vi "Measurement Logic.vi"() -> ()   [LabVIEW 2022 SP3, in "Frequency Response.lvlib"]
uses:
  Frequency Response.lvlib
  <vilib>/Plug-In SDKs/Measurements/Measure Call Context/Measure Call Context.lvclass
  Measurement Configuration.ctl
  shared/controls/sweep profile.ctl
  Measurement Results.ctl
  <vilib>/PDM Acquisition Toolkit/host/Classes/Tasks/PDM Tasks/Controls/Acquisition Mode.ctl
  <vilib>/PDM Acquisition Toolkit/shared/controls/clock mode.ctl
  shared/measurements/controls/units settings - mic.ctl
  shared/measurements/controls/measurement units.ctl
  shared/measurements/controls/single tone microphone measurement settings.ctl
  <vilib>/addons/_NISVFA/_Generation/Signal Generation/SV Signal/SV Signal.lvclass/SV Signal.ctl
  <vilib>/addons/_NISVFA/_Generation/Signal Generation/SV Discrete Sweep/SV Discrete Sweep.lvclass/SV Discrete Sweep.ctl
  <vilib>/addons/_NISVFA/_Generation/Signal Generation/SV Signal/Write Leading Synchronization Pulse Enable.vi
  <vilib>/addons/_NISVFA/_Generation/Signal Generation/SV Signal/Write Synchronization Pulse Duration.vi
  <vilib>/addons/_NISVFA/_Generation/Signal Generation/SV Signal/Write Synchronization Pulse Level.vi
  <vilib>/addons/_NISVFA/_Generation/Signal Generation/SV Signal/Write Synchronization Pulse Type.vi
  <vilib>/addons/_NISVFA/_Generation/Signal Generation/SV Signal/Read Total Samples.vi
  shared/measurements/sound and vibration/Align Waveforms by Leading Sync Pulse.vi
  <vilib>/addons/_NISVFA/_Generation/Signal Generation/SV Signal/Read Synchronization Pulse Waveform.vi
  <vilib>/addons/_NISVFA/_Shared subVIs/Common/svc_Check for Waveform Parameter Continuity (N Ch).vi
  Program Files/NI/LVAddons/nisvt/1/examples/Sound and Vibration/Audio Measurements/subVIs/sv_Append Virtual Reference.vi
  <vilib>/addons/_NISVFA/_Generation/Signal Generation/SV Discrete Sweep/Read Frequencies and Amplitudes.vi
  <vilib>/addons/_NISVFA/_Generation/Signal Generation/SV Signal/Calculate Number of Remaining Samples.vi
  shared/measurements/sound and vibration/Measure Delay for Active and Idle Channels.vi
  <vilib>/addons/_NISVFA/_Generation/Signal Generation/SV Signal/Read Leading Synchronization Pulse Enable.vi
  <vilib>/addons/_NISVFA/_Generation/Signal Generation/SV Signal/Read Trailing Synchronization Pulse Enable.vi
  <vilib>/addons/_NISVFA/_Shared subVIs/Common/svc_Check for Waveform Parameter Continuity (no state).vi
  <vilib>/addons/_NISVFA/_Shared subVIs/Common/sv_Get NI Property Name String.vi
  <vilib>/addons/Sound and Vibration/svt_Calibration/SV Measure Delay and Polarity and Coherence (Nx1).vi
  Program Files/NI/LVAddons/nisvt/1/examples/Sound and Vibration/Audio Measurements/subVIs/sv_Assign Delay to Idle Channels.vi
  <vilib>/addons/_NISVFA/_Shared subVIs/Common/svc_Get SV Channel Info.vi
  <vilib>/addons/Sound and Vibration/svt_Calibration/SV Measure Delay and Polarity and Coherence.vi
  <vilib>/addons/_NISVFA/_Shared subVIs/Common/svc_Unit Label to Engineering Units.vi
  <vilib>/addons/_NISVFA/_Shared subVIs/Common/svc_Engineering Units to Unit Label.vi
  <vilib>/Analysis/_algsub.llb/Vector Norm.vi
  <vilib>/Analysis/_algsub.llb/Real Vector Norm.vi
  <vilib>/addons/_NISVFA/_Shared subVIs/Common/SV Get Data Subset.vi
  <vilib>/addons/_NISVFA/_Shared subVIs/Common/svc_Get Array Subset (Index).vi
  <vilib>/addons/_NISVFA/_Shared subVIs/Common/svc_Coerce Index and Length.vi
  <vilib>/addons/_NISVFA/_Shared subVIs/Common/svc_Conditional Merge Error.vi
  <vilib>/addons/_NISVFA/_Generation/Signal Generation/SV Discrete Sweep/SV Discrete Sweep.lvclass
  C:/Program Files/NI/LVAddons/nisvt/1/vi.lib/addons/_NISVFA/_Generation/Signal Generation/SV Signal/SV Signal.lvclass
  C:/Program Files/NI/LVAddons/nisvt/1/vi.lib/addons/_NISVFA/_Generation/Signal Generation/SV Function/SV Function.lvclass
  <vilib>/addons/_NISVFA/_Generation/Signal Generation/SV Signal/Write Ramp Parameters.vi
  <vilib>/addons/_NISVFA/_Generation/Signal Generation/SV Signal/Write Measurement Duration.vi
  <vilib>/addons/_NISVFA/_Generation/Signal Generation/SV Function/Write Measurement Cycles.vi
  <vilib>/addons/_NISVFA/_Generation/Signal Generation/SV Signal/Write Pre-Measurement Settling Duration.vi
  <vilib>/addons/_NISVFA/_Generation/Signal Generation/SV Function/Write Pre-Measurement Settling Cycles.vi
  <vilib>/addons/_NISVFA/_Generation/Signal Generation/SV Signal/Write Sample Rate.vi
  <vilib>/addons/_NISVFA/_Generation/Signal Generation/SV Signal/Read Sample Rate.vi
  <vilib>/addons/_NISVFA/_Generation/Signal Generation/SV Signal/Read Generation State.vi
  <vilib>/addons/_NISVFA/_Generation/Signal Generation/SV Signal/Read System Timing Model.vi
  <vilib>/DAQmx/configure/timing.llb/DAQmx Timing (Sample Clock).vi
  <vilib>/DAQmx/miscellaneous.llb/DAQmx Fill In Error Info.vi
  <vilib>/addons/_NISVFA/_Generation/Signal Generation/SV Signal/Write System Timing Model.vi
  <vilib>/addons/_NISVFA/_Shared subVIs/Data Objects/Waveforms (DBL)/SV Read Newest Data.vi
  <vilib>/measure/maresamp.llb/Resample Waveforms (single shot).vi
  <vilib>/measure/maresamp.llb/Resample Waveform (single shot).vi
  <vilib>/addons/_NISVFA/_Shared subVIs/Common/svc_Check dt for Equal Sample Rates.vi
  <vilib>/Waveform/TSOps.llb/Timestamp Subtract.vi
  <vilib>/Analysis/2dsp.llb/CrossCorrelation.vi
  <vilib>/Analysis/2dsp.llb/1D Cross Correlation (DBL).vi
  <vilib>/addons/_NISVFA/_Shared subVIs/Common/svc_Fit Quadratic to Max Three Points in Array.vi
  <vilib>/Utility/error.llb/Error Cluster From Error Code.vi
  <vilib>/addons/_NISVFA/_Shared subVIs/Common/svc_Caller VI Returned in Error Source.vi
  <vilib>/addons/_NISVFA/_Shared subVIs/Common/SV Remove Delays (1,N) from Waveforms (N Ch) (DBL).vi
  <vilib>/addons/_NISVFA/_Shared subVIs/Common/SV Remove Delays from Waveforms.vi
  <vilib>/addons/_NISVFA/_Generation/Signal Generation/SV Signal/SV Signal.lvclass
  <vilib>/DAQmx/read.llb/DAQmx Read (Analog 1D Wfm NChan NSamp).vi
  <vilib>/addons/_NISVFA/_Generation/Signal Generation/SV Discrete Sweep/Configure Frequency Sweep at Constant Amplitude.vi
  <vilib>/addons/_NISVFA/_Shared subVIs/Data Objects/Waveforms (DBL)/SV Read Next Measurement Data.vi
  <vilib>/DAQmx/write.llb/DAQmx Write (Analog Wfm 1Chan NSamp).vi
  <vilib>/DAQmx/create/channels.llb/DAQmx Create Channel (AO-Voltage-Basic).vi
  <vilib>/DAQmx/configure/trigger.llb/DAQmx Start Trigger (Digital Edge).vi
  <vilib>/DAQmx/configure/events/hardwareSignals.llb/DAQmx Export Signal (Most Signals).vi
  <vilib>/DAQmx/create/channels.llb/DAQmx Create Channel (AI-Sound Pressure-Microphone).vi
  <vilib>/addons/_NISVFA/_Shared subVIs/Data Objects/Waveforms (DBL)/Waveforms (N Ch).lvclass
  <resource>/objmgr/daqmx.rc
  shared/combined digital api/Combo Digital Audio API.lvlib
  <vilib>/PDM Acquisition Toolkit/host/Classes/Tasks/PDM Tasks/PDM Task.lvclass
  <vilib>/PDM Acquisition Toolkit/shared/PDM Shared.lvlib
  C:/Program Files/NI/LVAddons/nisvt/1/vi.lib/addons/_NISVFA/_Generation/Signal Generation/SV Sinusoid/SV Sinusoid.lvclass
  C:/Program Files/NI/LVAddons/nisvt/1/vi.lib/addons/_NISVFA/_Generation/Signal Generation/SV Discrete Sweep/SV Discrete Sweep.lvclass
panel:
  out "alignment reference detected":bool
  in  "Tab Control":T1(tab)
  out "Waveform Graph":waveform(dbl)[](graph)=[{"t0"=timestamp(4.019687510148735 s since 1904-01-01), "dt"=2.0833333385932442e-05, "Y"=array[64206 elements], "attributes"=variant("NI_ChannelName"=variant(string "PDMI0L"))}, {"t0"=timestamp(3813245559.9758506 s since 1904-01-01), "dt"=2.083333332672055e-05, "Y"=array[64206 elements], "attributes"=variant("NI_ChannelName"=variant(string "PXI1Slot2/ai0"), "NI_UnitDescription"=variant(string "Pascals"), "NI_dBReference"=variant(dbl 2e-05))}]
  out "XY Graph":cluster{"X":dbl[], "Y":dbl[]}[](graph)=[{"X"=[10000.515193969344, 9302.18746152866, 8642.225793958956, 8072.5151484177995, 7517.135528017866, 6994.7900792599785, 6516.982892518442, 6058.424706212935, 5641.998588430436, 5250.318521955464, 4886.606525619628, 4570.492017550713, 4216.337677030385, 3948.807437432098, 3680.8618397757855, 3411.195823757008, 3175.8174592444034, 2964.339402263135, 2756.802808481013, 2567.086307416725, 2389.5560064921156, 2225.4908957208995, 2083.833386349876, 1930.3992531905435, 1795.6161670550198, 1671.2855279868957, 1555.4312030353315, 1448.6805749167713, 1348.0369547777334, 1254.9797896016998, 1167.9972818297738, 1087.7149037445288, 1012.7049452021939, 943.0827780385741, 878.1558990917348, 816.9001564834517, 760.7276526170439, 708.052836443301, 659.2337132846405, 613.081846735373, 571.0033254400446, 531.7294307990026, 495.4768426445635, 460.79511341572686, 429.1046086454286, 399.4701284346599, 371.8774839415845, 346.2729235864874, 322.5427149186949, 300.0056069768776], "Y"=[106.24290251289379, 100.6726523123771, 101.64552994870905, 106.01173398447203, 104.36678448317771, 100.73388716799067, 99.33351948245948, 95.06365915809951, 95.3500686342148, 93.48892064011515, 88.4034433059791, 90.75216149582737, 94.99452438129994, 99.80747932171317, 100.55760031357137, 98.71429283890593, 98.87757947282614, 100.11015017403336, 99.49448006964708, 100.67096957410372, 100.30830119783818, 98.9841022091353, 98.54908592521276, 98.62715495892607, 97.20797644231718, 95.67322241840984, 95.01533802784917, 95.66376864277066, 97.07828478757129, 97.10876590792577, 95.67172372656144, 93.85226917638678, 91.93460327856648, 90.69215854367033, 89.98405175411321, 90.0570504454669, 89.76614225050021, 89.43829950832733, 88.92234495571091, 87.14179662323579, 87.29122881703591, 87.5780835733913, 87.42071486917925, 87.78757177238776, 87.79439239227699, 86.62918319323236, 84.89697341828975, 82.48376663209544, 77.07716014579213, 82.45870427224955]}, {"X"=[10000.515193969344, 9302.18746152866, 8642.225793958956, 8072.5151484177995, 7517.135528017866, 6994.7900792599785, 6516.982892518442, 6058.424706212935, 5641.998588430436, 5250.318521955464, 4886.606525619628, 4570.492017550713, 4216.337677030385, 3948.807437432098, 3680.8618397757855, 3411.195823757008, 3175.8174592444034, 2964.339402263135, 2756.802808481013, 2567.086307416725, 2389.5560064921156, 2225.4908957208995, 2083.833386349876, 1930.3992531905435, 1795.6161670550198, 1671.2855279868957, 1555.4312030353315, 1448.6805749167713, 1348.0369547777334, 1254.9797896016998, 1167.9972818297738, 1087.7149037445288, 1012.7049452021939, 943.0827780385741, 878.1558990917348, 816.9001564834517, 760.7276526170439, 708.052836443301, 659.2337132846405, 613.081846735373, 571.0033254400446, 531.7294307990026, 495.4768426445635, 460.79511341572686, 429.1046086454286, 399.4701284346599, 371.8774839415845, 346.2729235864874, 322.5427149186949, 300.0056069768776], "Y"=[91.64090515498991, 89.41151069171059, 92.04741888067618, 94.56853414486562, 97.11782992067077, 95.49243172718333, 94.15152648147392, 95.32102047134535, 95.5110270658068, 95.86352291824593, 93.17672927225416, 91.61193802219867, 93.35925871582867, 93.51937158432973, 93.06610584193339, 90.15357116773417, 81.84029984961566, 88.75078558356509, 93.20005221332694, 92.54289378947331, 91.78015992589373, 88.22724272956208, 88.65309856779227, 88.77157262510818, 89.79924341832859, 91.42003698720545, 92.03446484373595, 91.53102414111623, 91.8372179753682, 93.12393536277025, 93.85412628778221, 94.30397033683798, 93.9977062320192, 92.95587820092351, 92.65066740508803, 92.58936410631237, 92.26042392173126, 91.62651844421018, 91.01102372338258, 89.94642482302169, 90.36007289091827, 90.94921636953995, 90.9179558226102, 91.33466472788919, 91.68652532539937, 91.49970769995883, 90.95792273818724, 91.04350130520892, 90.35207361093349, 90.71889644946252]}, {"X"=[10000.515193969344, 9302.18746152866, 8642.225793958956, 8072.5151484177995, 7517.135528017866, 6994.7900792599785, 6516.982892518442, 6058.424706212935, 5641.998588430436, 5250.318521955464, 4886.606525619628, 4570.492017550713, 4216.337677030385, 3948.807437432098, 3680.8618397757855, 3411.195823757008, 3175.8174592444034, 2964.339402263135, 2756.802808481013, 2567.086307416725, 2389.5560064921156, 2225.4908957208995, 2083.833386349876, 1930.3992531905435, 1795.6161670550198, 1671.2855279868957, 1555.4312030353315, 1448.6805749167713, 1348.0369547777334, 1254.9797896016998, 1167.9972818297738, 1087.7149037445288, 1012.7049452021939, 943.0827780385741, 878.1558990917348, 816.9001564834517, 760.7276526170439, 708.052836443301, 659.2337132846405, 613.081846735373, 571.0033254400446, 531.7294307990026, 495.4768426445635, 460.79511341572686, 429.1046086454286, 399.4701284346599, 371.8774839415845, 346.2729235864874, 322.5427149186949, 300.0056069768776], "Y"=[16.70136574753728, 13.360510010299905, 11.697479457666276, 13.542568229239805, 9.348322952140336, 7.340823830440741, 7.281361390618955, 1.842007076387561, 1.9384099580413912, -0.2752338884973815, -2.67391757664167, 1.2395918632620928, 3.7346340551046646, 8.38747612701684, 9.590862861271376, 10.66009006080516, 19.136648012843878, 13.458732980101672, 8.393796245953538, 10.227444174263809, 10.627509661577847, 12.85622786920662, 11.995355747053893, 11.95495072345129, 9.508101413621986, 6.352553820837785, 5.08024157374662, 6.232112891287827, 7.340435201836486, 6.084198934788916, 3.9169658284126294, 1.647667229182205, 0.03626543618068556, -0.1643512676197778, -0.5672472613414206, -0.43294527121207604, -0.3949132815976517, -0.08885054624944555, 0.010689621961732065, -0.705259810152497, -0.9694756842489616, -1.271764406515259, -1.3978725637975478, -1.447724565868028, -1.7927645434889845, -2.77115611709307, -3.9615809302640903, -6.4603662834800835, -11.175545075507955, -6.160823787579573]}]
  out "Distortion":cluster{"X":dbl[], "Y":dbl[]}[](graph)=[{"X"=[10000.515193969344, 9302.18746152866, 8642.225793958956, 8072.5151484177995, 7517.135528017866, 6994.7900792599785, 6516.982892518442, 6058.424706212935, 5641.998588430436, 5250.318521955464, 4886.606525619628, 4570.492017550713, 4216.337677030385, 3948.807437432098, 3680.8618397757855, 3411.195823757008, 3175.8174592444034, 2964.339402263135, 2756.802808481013, 2567.086307416725, 2389.5560064921156, 2225.4908957208995, 2083.833386349876, 1930.3992531905435, 1795.6161670550198, 1671.2855279868957, 1555.4312030353315, 1448.6805749167713, 1348.0369547777334, 1254.9797896016998, 1167.9972818297738, 1087.7149037445288, 1012.7049452021939, 943.0827780385741, 878.1558990917348, 816.9001564834517, 760.7276526170439, 708.052836443301, 659.2337132846405, 613.081846735373, 571.0033254400446, 531.7294307990026, 495.4768426445635, 460.79511341572686, 429.1046086454286, 399.4701284346599, 371.8774839415845, 346.2729235864874, 322.5427149186949, 300.0056069768776], "Y"=[16.217727310705225, 20.84074917090225, 16.195429434202673, 9.432271439835473, 8.60044368770178, 8.519063186768467, 13.210861864452017, 27.492164349040205, 21.58790677839547, 23.99872485014149, 43.08008579200741, 39.82453976197276, 26.29483237696651, 10.41992140081969, 12.149453076906052, 16.58141797816388, 7.456261102076903, 8.18939536410412, 9.378984922736786, 6.459938026885411, 5.625002912452868, 6.709745306696694, 8.06364104767742, 4.143469371298831, 9.941832586386624, 6.511469455605076, 8.24578057644499, 7.133488127015056, 7.948278482892307, 5.918137330973101, 7.686132098075285, 8.192360492558969, 4.614308882077067, 10.193621277155048, 13.713114417022911, 12.30586404412293, 17.65240676946193, 12.268613530400762, 16.282891580937743, 21.245666734699874, 17.94412066197058, 12.191433903206923, 14.370812815144424, 10.92835019259563, 5.808657086467276, 9.926401045918213, 12.376918047099633, 10.165684026803588, 31.404399742161225, 12.894742349029942]}, {"X"=[10000.515193969344, 9302.18746152866, 8642.225793958956, 8072.5151484177995, 7517.135528017866, 6994.7900792599785, 6516.982892518442, 6058.424706212935, 5641.998588430436, 5250.318521955464, 4886.606525619628, 4570.492017550713, 4216.337677030385, 3948.807437432098, 3680.8618397757855, 3411.195823757008, 3175.8174592444034, 2964.339402263135, 2756.802808481013, 2567.086307416725, 2389.5560064921156, 2225.4908957208995, 2083.833386349876, 1930.3992531905435, 1795.6161670550198, 1671.2855279868957, 1555.4312030353315, 1448.6805749167713, 1348.0369547777334, 1254.9797896016998, 1167.9972818297738, 1087.7149037445288, 1012.7049452021939, 943.0827780385741, 878.1558990917348, 816.9001564834517, 760.7276526170439, 708.052836443301, 659.2337132846405, 613.081846735373, 571.0033254400446, 531.7294307990026, 495.4768426445635, 460.79511341572686, 429.1046086454286, 399.4701284346599, 371.8774839415845, 346.2729235864874, 322.5427149186949, 300.0056069768776], "Y"=[0.0, 0.25312800975628047, 0.8952288719354575, 0.31008590575295464, 0.42591094258016393, 0.6544716506371486, 1.750113903331441, 5.903117592157415, 6.84718385189155, 3.853898957210377, 9.715834139386475, 8.4492715545514, 5.416876106708672, 2.439875465825829, 2.7749898561584527, 2.567597223711487, 1.1463848704096056, 1.0105020564798335, 1.3968968391130572, 1.238267035899352, 1.1087284101949968, 1.248061767835907, 0.6904720885061408, 0.7000682530992854, 0.7731022091918685, 0.7592672659672433, 1.080836118646896, 0.7899620817383691, 0.6548737988955111, 0.7118382718922972, 0.7060653395482884, 0.9264165916141978, 1.187105642509263, 1.1625527620168528, 1.0146790377003432, 1.0212901318036687, 0.7917558334265945, 1.0614960396916668, 0.9714495220749704, 0.9660479736684572, 1.0463172231210063, 1.1730608288814786, 1.1284424274903213, 0.9628257682012435, 1.038672486680222, 1.1566657977473211, 1.3697348199716954, 2.2035320325702292, 3.332813527629286, 2.0395970822026435]}]
  out "measurement results":T2={"channel name"="Empty", "frequency (Hz)"=[0.0], "amplitude (dBr)"=[0.0], "THD+N"=[0.0], "THD"=[0.0], "wfm - dt"=0.0, "wfm - data"=[0.0], "ref mic wfm - dt"=0.0, "ref mic wfm - data"=[0.0]}
  in  "measurement configuration":T3={"digital channel list"="PXI1Slot5\\PDMi 0L", "input cfg file"="C:\\dev\\digital-microphone\\test\\test-PDM.inputcfg", "digital mic sensitivity (dBFS)"=-26.0, "ref mic channel"="PXI1Slot2/ai0", "ref mic sensitivity (mV/Pa)"=50.0, "output channel"="PXI1Slot2/ao0", "output level (dBSPL)"=94.0, "output voltage ratio"=4.25, "start frequency"=20000.0, "stop frequency"=100.0, "number of steps"=100.0, "sweep profile"=enum."Linear", "min measurement cycles"=20, "min measurement time (s)"=0.1, "min settling cycles"=0, "min settling time (s)"=0.0} {"number of steps" format="%#_13g"; "start frequency" format="%#_13g"; "output voltage ratio" format="%#.3f"; "digital mic sensitivity (dBFS)" format="%#_13g"}
  out "measure call context out":refnum<class "Measure Call Context.lvclass">
  in  "measure call context in":refnum<class "Measure Call Context.lvclass">
  out "error out":errorcluster
  in  "error in":errorcluster
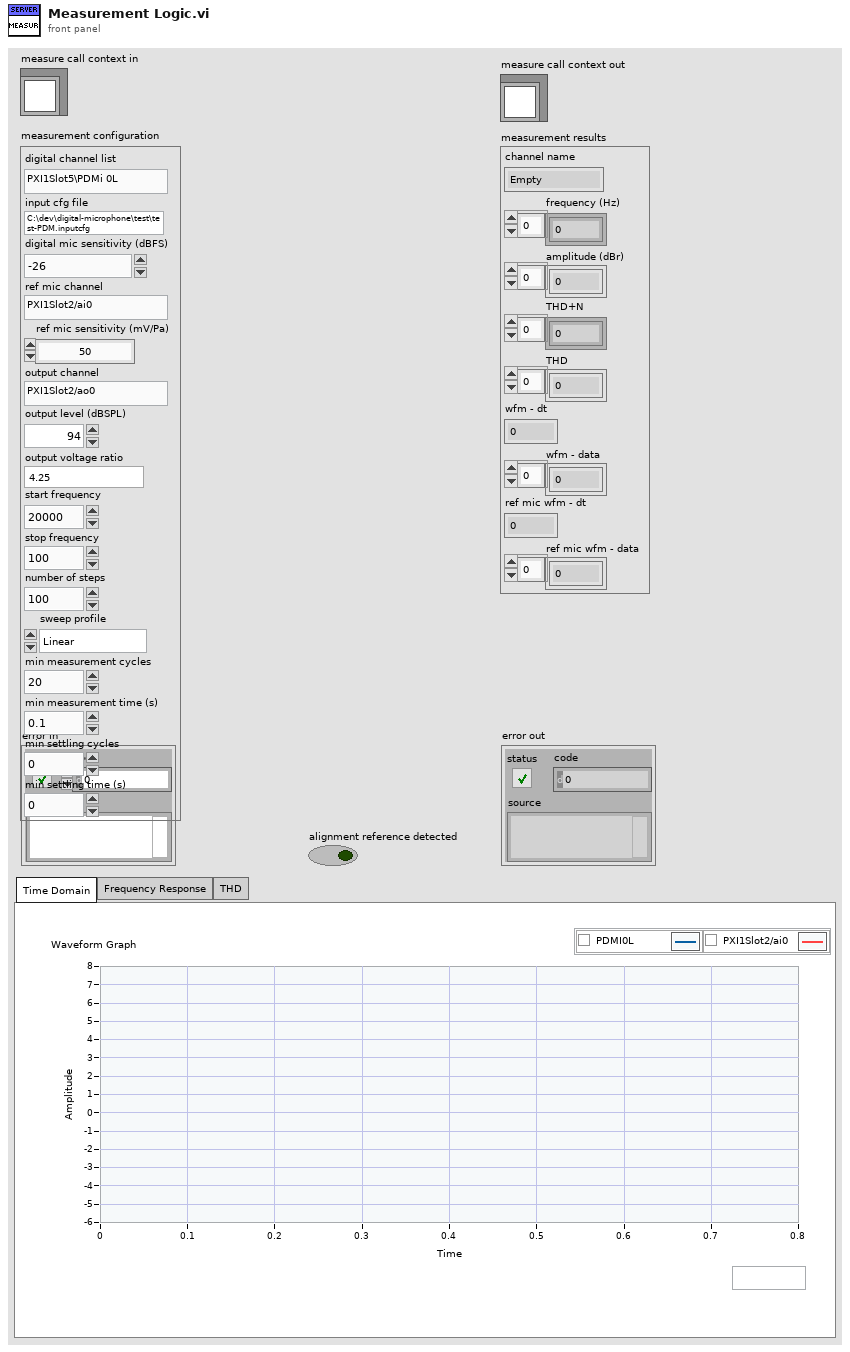
[diagram p1: front panel]
types:
  T1 = enum32{"Time Domain", "Frequency Response", "THD"}
  T2 = typedef "Frequency Response.lvlib/Measurement Results.ctl" = cluster{"channel name":string, "frequency (Hz)":dbl[], "amplitude (dBr)":dbl[], "THD+N":dbl[], "THD":dbl[], "wfm - dt":dbl, "wfm - data":dbl[], "ref mic wfm - dt":dbl, "ref mic wfm - data":dbl[]}
  T3 = typedef "Frequency Response.lvlib/Measurement Configuration.ctl" = cluster{"digital channel list":string, "input cfg file":string, "digital mic sensitivity (dBFS)":dbl, "ref mic channel":string, "ref mic sensitivity (mV/Pa)":dbl, "output channel":string, "output level (dBSPL)":dbl, "output voltage ratio":dbl, "start frequency":dbl, "stop frequency":dbl, "number of steps":dbl, "sweep profile":T4, "min measurement cycles":u32, "min measurement time (s)":dbl, "min settling cycles":u32, "min settling time (s)":dbl}
  T4 = typedef "sweep profile.ctl" = enum32{"Linear", "Logarithmic"}
  T5 = enum16{"Noise", "MLS", "Chirp", "Monopulse", "Custom"}
  T6 = typedef "PDM Shared.lvlib/clock mode.ctl" = enum16{"divided clock", "DDS"}
  T7 = typedef "PDM Acquisition Class Library.lvlib/PDM Task.lvclass/Acquisition Mode.ctl" = enum16{"Finite", "Continuous"}
  T8 = cluster{"profile":enum16{"Linear", "Half cosine"}, "durations [s]":cluster{"ramp-up":dbl, "transition":dbl, "ramp-down":dbl}}
  T9 = typedef "Combo Digital Audio API.lvlib/task.ctl" = cluster{"task ref":u64, "audio type":T10, "sample rate":dbl}
  T10 = typedef "input type.ctl" = enum32{"Digital Serial", "PDM"}
  T11 = cluster{"frequency [Hz]":dbl, "amplitude [V]":dbl}[]
  T12 = typedef "single tone microphone measurement settings.ctl" = cluster{"Band start":dbl, "Band stop":dbl, "Frequency":dbl}
  T13 = typedef "units settings - mic.ctl" = cluster{"SNR units":T14, "THD+N units":T14, "THD units":T14}
  T14 = typedef "measurement units.ctl" = enum32{"dB", "%", "x/y"}
  T15 = typedef "single tone microphone measurements.ctl" = cluster{"channel":string, "frequency (Hz)":dbl, "amplitude (Pa rms)":dbl, "amplitude (dBSPL)":dbl, "SNR":dbl, "THD+N":dbl, "THD":dbl, "phase (deg)":dbl}
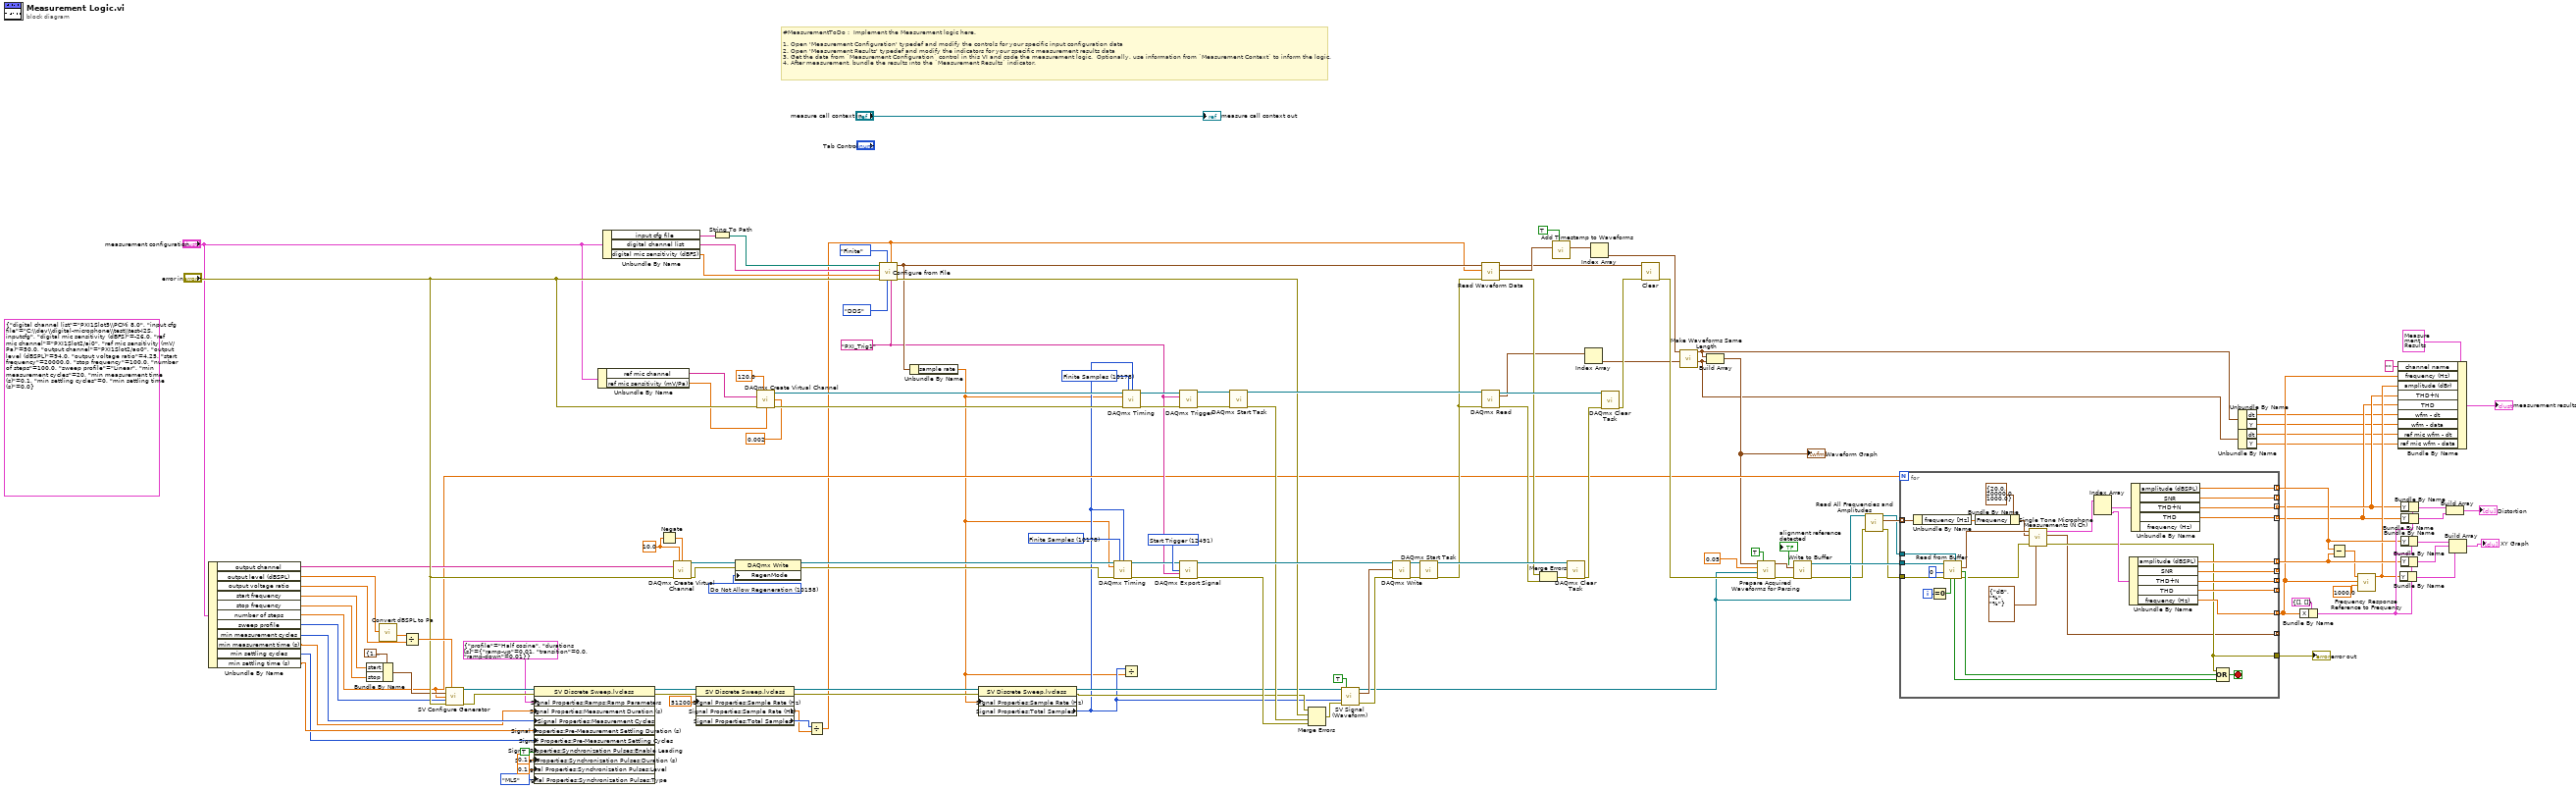
[diagram p0: block diagram]
diagram:
  (unwired) T3 {"digital channel list"="PXI1Slot5\\PCMi 8.0", "input cfg file"="C:\\dev\\digital-microphone\\test\\test-I2S.inputcfg", "digital mic sensitivity (dBFS)"=-26.0, "ref mic channel"="PXI1Slot2/ai0", "ref mic sensitivity (mV/Pa)"=50.0, "output channel"="PXI1Slot2/ao0", "output level (dBSPL)"=94.0, "output voltage ratio"=4.25, "start frequency"=20000.0, "stop frequency"=100.0, "number of steps"=100.0, "sweep profile"=enum."Linear", "min measurement cycles"=20, "min measurement time (s)"=0.1, "min settling cycles"=0, "min settling time (s)"=0.0} ("measurement configuration 2")
  w52 = "PXI_Trig1"
  w97 = 10178 items=["Finite Samples"=10178, "Continuous Samples"=10123, "Hardware Timed Single Point"=12522] ("sample mode")
  w106 = 12491 items=["AI Convert Clock"=12484, "10MHz Reference Clock"=12536, "20MHz Timebase Clock"=12486, "Sample Clock"=12487, "Advance Trigger"=12488, "Reference Trigger"=12490, "Start Trigger"=12491, "Advance Complete Event"=12492, "AI Hold Complete Event"=12493, "Counter Output Event"=12494, "Change Detection Event"=12511, "Watchdog Timer Expired Event"=12512] ("signal")
  w126 = 10158 items=["Allow Regeneration"=10097, "Do Not Allow Regeneration"=10158] ("RegenMode")
  w128 = 10.0 ("maximum value")
  w129 = 10178 items=["Finite Samples"=10178, "Continuous Samples"=10123, "Hardware Timed Single Point"=12522] ("sample mode")
  # "#MeasurementToDo :  Implement the Measurement logic here.\n\n1. Open 'Measurement Configuration' typedef and modify the controls for your specific input configuration data\n2. Open 'Measurement Results' typedef and modify the indicators for your specific measurement results data\n3. Get the data from `Measurement Configuration` control in this VI and code the measurement logic.  Optionally, use information from `Measurement Context` to inform the logic.\n4. After measurement, bundle the results into the `Measurement Results` indicator."
  n1 = Unbundle By Name("measurement configuration") -> ("output channel"=w47:string, "output level (dBSPL)"=w46:dbl, "output voltage ratio"=w45:dbl, "start frequency"=w42:dbl, "stop frequency"=w41:dbl, "number of steps"=w40:dbl, "sweep profile"=w39:T4, "min measurement cycles"=w4:u32, "min measurement time (s)"=w3:dbl, "min settling cycles"=w1:u32, "min settling time (s)"=w2:dbl)
  n2 = Bundle By Name(cluster=cluster{"start":dbl, "stop":dbl} {"start"=10000.0, "stop"=300.0} ("sweep range"), "start"=w42, "stop"=w41) -> (w43:cluster{"start":dbl, "stop":dbl})
  n3 = call "Convert dBSPL to Pa.vi"("dB SPL"=w46) -> ("Pa pk"=w107:dbl)  [unwired: 9 in, 1 out]
  n4 = Divide(x=w107, y=w45) -> (x/y=w130:dbl)
  n5 = call-poly <vilib>:"SV Configure Generator.vi"("amplitude"=w130, "frequency range [Hz]"=w43, "number of steps"=w40, "profile"=w39, "error in (no error)"="error in") -> ("signal configuration"=w132:refnum<class "SV Discrete Sweep.lvclass">, "error out"=w131:errorcluster)  [unwired: 9 in]
  n6 = property class="SV Discrete Sweep.lvclass"(reference=w132, error in=w131, "Signal Properties:Ramps:Ramp Parameters"=T8 {"profile"=enum."Half cosine", "durations [s]"={"ramp-up"=0.01, "transition"=0.0, "ramp-down"=0.01}} ("Ramp Parameters"), "Signal Properties:Measurement Duration (s)"=w3, "Signal Properties:Measurement Cycles"=w4, "Signal Properties:Pre-Measurement Settling Duration (s)"=w2, "Signal Properties:Pre-Measurement Settling Cycles"=w1, "Signal Properties:Synchronization Pulses:Enable Leading"=TRUE ("Synchronization Pulses:Enable Leading"), "Signal Properties:Synchronization Pulses:Duration (s)"=0.1 ("Synchronization Pulses:Duration"), "Signal Properties:Synchronization Pulses:Level"=0.1 ("Synchronization Pulses:Level"), "Signal Properties:Synchronization Pulses:Type"=T5."MLS" ("Synchronization Pulses:Type")) -> (reference out=w119:refnum<class "SV Discrete Sweep.lvclass">, error out=w120:errorcluster)
  n7 = Unbundle By Name("measurement configuration") -> ("ref mic channel"=w49:string, "ref mic sensitivity (mV/Pa)"=w48:dbl)
  n8 = Unbundle By Name("measurement configuration") -> ("input cfg file"=w71:string, "digital channel list"=w69:string, "digital mic sensitivity (dBFS)"=w66:dbl)
  n9 = Negate(x=w128) -> (-x=w127:dbl)
  n10 = call-poly <vilib>:"DAQmx Create Virtual Channel.vi"("maximum value"=w128, "minimum value"=w127, "physical channels"=w47, "error in"="error in") -> ("task out"=w125:refnum<k21>, "error out"=w123:errorcluster)  [unwired: 10 in]
  n11 = property on="Property Node" class="SV Discrete Sweep.lvclass"(reference=w119, error in=w120, "Signal Properties:Sample Rate (Hz)"=51200.0 ("Sample Rate (Hz)")) -> (reference out=w55:refnum<class "SV Discrete Sweep.lvclass">, error out=w54:errorcluster, "Signal Properties:Sample Rate (Hz)"=w10:dbl, "Signal Properties:Total Samples"=w58:i32)
  n12 = String To Path(string=w71) -> (path=w70:path)
  n13 = property class="DAQmx Write"(reference=w125, error in=w123, "RegenMode"=w126) -> (reference out=w124:refnum<k21>, error out=w122:errorcluster)
  n14 = call-poly <vilib>:"DAQmx Create Virtual Channel.vi"("maximum sound pressure level"=120.0, "physical channels"=w49, "current excitation value"=0.002, "error in"="error in", "microphone sensitivity"=w48) -> ("task out"=w99:refnum<k21>, "error out"=w98:errorcluster)  [unwired: 9 in]
  n15 = Divide(x=w58, y=w10) -> (x/y=w38:dbl)
  n16 = call "Configure from File.vi"("digital trigger"=w52, "acq duration (s)"=w38, "clock mode"=clock_mode."DDS", "acquisition mode"=Acquisition_Mode."Finite", "error in (no error)"="error in", "microphone sensitivity (dBFS)"=w66, "channels"=w69, "file path"=w70) -> ("error out"=w62:errorcluster, "task"=w56:T9)  [unwired: 2 in]
  n17 = Unbundle By Name(w56) -> ("sample rate"=w11:dbl)
  n18 = property on="Property Node" class="SV Discrete Sweep.lvclass"(reference=w55, error in=w54, "Signal Properties:Sample Rate (Hz)"=w11) -> (reference out=w53:refnum<class "SV Discrete Sweep.lvclass">, error out=w51:errorcluster, "Signal Properties:Total Samples"=w12:i32)
  n19 = call-poly <vilib>:"DAQmx Timing.vi"("task/channels in"=w124, "sample mode"=w129, "samples per channel"=w12, "rate"=w11, "error in"=w122) -> ("task out"=w103:refnum<k21>, "error out"=w102:errorcluster)  [unwired: 9 in]
  n20 = call-poly <vilib>:"DAQmx Timing.vi"("task/channels in"=w99, "sample mode"=w97, "samples per channel"=w12, "rate"=w11, "error in"=w98) -> ("task out"=w94:refnum<k21>, "error out"=w93:errorcluster)  [unwired: 9 in]
  n21 = Divide(x=w12, y=w11) -> ()  [unwired: 1 out]
  n22 = call-poly <vilib>:"DAQmx Export Signal.vi"("task/channels in"=w103, "signal"=w106, "output terminal"=w52, "error in"=w102) -> ("task out"=w105:refnum<k21>, "error out"=w104:errorcluster)  [unwired: 10 in]
  n23 = call-poly <vilib>:"DAQmx Trigger.vi"("task/channels in"=w94, "source"=w52, "error in"=w93) -> ("task out"=w91:refnum<k21>, "error out"=w92:errorcluster)  [unwired: 11 in]
  n24 = call <vilib>:"DAQmx Start Task.vi"("task/channels in"=w91, "error in"=w92) -> ("task out"=w89:refnum<k21>, "error out"=w90:errorcluster)  [unwired: 12 in]
  n25 = Merge Errors(w51, w62, w90, w104) -> (w117:errorcluster)
  n26 = call-dynamic "SV Signal (Waveform).vi"("signal configuration"=w53, "reset"=TRUE, "samples"=w12, "error in (no error)"=w117) -> ("signal configuration"=w34:refnum<class "SV Discrete Sweep.lvclass">, "output waveform"=w115:waveform(dbl), "error out"=w116:errorcluster)  [unwired: 6 in, 3 out]
  n27 = call-poly <vilib>:"DAQmx Write.vi"("task/channels in"=w105, "data"=w115, "error in"=w116) -> ("task out"=w113:refnum<k21>, "error out"=w114:errorcluster)  [unwired: 10 in, 1 out]
  n28 = call <vilib>:"DAQmx Start Task.vi"("task/channels in"=w113, "error in"=w114) -> ("task out"=w112:refnum<k21>, "error out"=w65:errorcluster)  [unwired: 12 in]
  n29 = call "Read Waveform Data.vi"("error in (no error)"=w65, "acq duration (s)"=w38, "task"=w56) -> ("error out"=w64:errorcluster, "waveforms"=w63:waveform(dbl)[], "task"=w61:T9)  [unwired: 6 in]
  n30 = call-poly <vilib>:"DAQmx Read.vi"("task/channels in"=w89, "error in"=w65) -> ("task out"=w88:refnum<k21>, "data"=w19:waveform(dbl)[], "error out"=w85:errorcluster)  [unwired: 11 in]
  n31 = Merge Errors(w64, w85) -> (w86:errorcluster)
  n32 = call "Add Timestamp to Waveforms.vi"("initialize"=TRUE, "waveforms"=w63) -> ("waveforms"=w18:waveform(dbl)[])  [unwired: 9 in]
  n33 = call <vilib>:"DAQmx Clear Task.vi"("task in"=w112, "error in"=w86) -> ("error out"=w87:errorcluster)  [unwired: 13 in]
  n34 = Index Array(array=w19) -> (element=w8:waveform(dbl))  [unwired: 1 in]
  n35 = Index Array(array=w18) -> (element=w6:waveform(dbl))  [unwired: 1 in]
  n36 = call <vilib>:"DAQmx Clear Task.vi"("task in"=w88, "error in"=w87) -> ("error out"=w60:errorcluster)  [unwired: 13 in]
  n37 = call "Clear.vi"("error in (no error)"=w60, "task"=w61) -> ("error out"=w59:errorcluster)  [unwired: 9 in]
  n38 = call "Make Waveforms Same Length.vi"("waveform 2"=w8, "waveform 1"=w6) -> ("waveform 2"=w7:waveform(dbl), "waveform 1"=w5:waveform(dbl))  [unwired: 8 in]
  n39 = Build Array(w5, w7) -> (w28:waveform(dbl)[])
  "Waveform Graph" <- w28
  n40 = call "Prepare Acquired Waveforms for Parsing.vi"("restart (F)"=TRUE, "error in"=w59, "SV Signal"=w34, "tolerance"=0.05, "acquired channel waveforms"=w28) -> ("error out"=w110:errorcluster, "aligned channel waveforms"=w84:waveform(dbl)[], "alignment reference detected"=→"alignment reference detected":bool)  [unwired: 4 in]
  n41 = call <vilib>:"Write to Buffer.vi"("error in (no error)"=w110, "waveforms"=w84) -> ("error out"=w32:errorcluster, "buffer out"=w109:refnum<data-value>)  [unwired: 7 in, 1 out]
  n42 = call <vilib>:"Read All Frequencies and Amplitudes.vi"("error in (no error)"=w32, "signal configuration"=w34) -> ("error out"=w31:errorcluster, "frequencies and amplitudes"=w33:T11, "signal configuration"=w30:refnum<class "SV Discrete Sweep.lvclass">)  [unwired: 7 in]
  n43 = for {
    N: w40 -> [_]
    tunnel: w109 -> [w161]
    tunnel: w30 -> [w160]
    tunnel: w31 -> [w159]
    tunnel: [w143] -> w24 mode=indexing
    tunnel: [w144] -> w74 mode=indexing
    tunnel: [w151] -> w73 mode=indexing
    tunnel: [w150] -> _ mode=indexing
    tunnel: [w149] -> w22 mode=indexing
    tunnel: [w148] -> w21 mode=indexing
    tunnel: [w142] -> _ mode=indexing
    tunnel: [w141] -> _ mode=indexing
    tunnel: [w140] -> _ mode=indexing
    tunnel: [w139] -> w50
    tunnel: [w138] -> _ mode=indexing
    tunnel: w33 -> [w135] mode=indexing
    i -> [w156]
    stop <- w157 stop-if-true
    n44 = Unbundle By Name(w135) -> ("frequency [Hz]"=w134:dbl)
    n45 = Equal To 0?(x=w156) -> (x = 0?=w155:bool)
    n46 = call-poly <vilib>:"Read from Buffer.vi"("test signal configuration"=w160, "reset start (F)"=w155, "error in (no error)"=w159, "timeout (1000 ms)"=0, "buffer"=w161) -> ("error out"=w154:errorcluster, "end of buffer"=w158:bool, "waveforms subset"=w146:waveform(dbl)[], "done"=w163:bool)  [unwired: 2 in, 1 out]
    n47 = Bundle By Name(cluster=T12 {"Band start"=20.0, "Band stop"=20000.0, "Frequency"=1000.0} ("measurement settings"), "Frequency"=w134) -> (w137:T12)
    n48 = call "Single Tone Microphone Measurements (N Ch).vi"("units settings"=T13 {"SNR units"=enum."dB", "THD+N units"=enum."%", "THD units"=enum."%"}, "error in"=w154, "measurement settings"=w137, "waveforms"=w146) -> ("error out"=w139:errorcluster, "waveforms"=w138:waveform(dbl)[], "measurements"=w153:T15[])  [unwired: 4 in, 1 out]
    n49 = Index Array(array=w153) -> (element #1=w152:T15, element #2=w145:T15)  [unwired: 2 in]
    n50 = Unbundle By Name(w145) -> ("amplitude (dBSPL)"=w144:dbl, "SNR"=w140:dbl, "THD+N"=w141:dbl, "THD"=w142:dbl, "frequency (Hz)"=w143:dbl)
    n51 = Unbundle By Name(w152) -> ("amplitude (dBSPL)"=w151:dbl, "SNR"=w150:dbl, "THD+N"=w149:dbl, "THD"=w148:dbl)  [unwired: 1 out]
    n52 = Compound Arithmetic op=OR(w139, w158, w163) -> (w157:bool)
  }
  "error out" <- w50
  n53 = Unbundle By Name(w5) -> ("dt"=w17:dbl, "Y"=w14:dbl[])
  n54 = Unbundle By Name(w7) -> ("dt"=w16:dbl, "Y"=w13:dbl[])
  n55 = Bundle By Name(cluster=cluster{"X":dbl[], "Y":dbl[]} {"X"=[], "Y"=[]} ("THD vs Amplitude"), "X"=w24) -> (w75:cluster{"X":dbl[], "Y":dbl[]})
  n56 = Subtract(x=w73, y=w74) -> (x-y=w72:dbl[])
  n57 = call "Frequency Response Reference to Frequency.vi"("reference frequency"=1000.0, "frequency"=w24, "amplitude (dBPL)"=w72) -> ("amplitude (dBr)"=w23:dbl[])  [unwired: 8 in]
  n58 = Bundle By Name(cluster=T2 {"channel name"="Empty", "frequency (Hz)"=[0.0], "amplitude (dBr)"=[0.0], "THD+N"=[0.0], "THD"=[0.0], "wfm - dt"=0.0, "wfm - data"=[0.0], "ref mic wfm - dt"=0.0, "ref mic wfm - data"=[0.0]} ("measurement results"), "channel name"="", "frequency (Hz)"=w24, "amplitude (dBr)"=w23, "THD+N"=w22, "THD"=w21, "wfm - dt"=w17, "wfm - data"=w14, "ref mic wfm - dt"=w16, "ref mic wfm - data"=w13) -> (→"measurement results":T2)
  n59 = Bundle By Name(cluster=w75, "Y"=w23) -> (w76:cluster{"X":dbl[], "Y":dbl[]})
  n60 = Bundle By Name(cluster=w75, "Y"=w73) -> (w81:cluster{"X":dbl[], "Y":dbl[]})
  n61 = Bundle By Name(cluster=w75, "Y"=w74) -> (w83:cluster{"X":dbl[], "Y":dbl[]})
  n62 = Bundle By Name(cluster=w75, "Y"=w22) -> (w80:cluster{"X":dbl[], "Y":dbl[]})
  n63 = Bundle By Name(cluster=w75, "Y"=w21) -> (w79:cluster{"X":dbl[], "Y":dbl[]})
  n64 = Build Array(w80, w79) -> (→"Distortion":cluster{"X":dbl[], "Y":dbl[]}[])
  n65 = Build Array(w81, w83, w76) -> (→"XY Graph":cluster{"X":dbl[], "Y":dbl[]}[])
  "measure call context out" <- "measure call context in"
